vi "10_Scope.vi"(8 "error in (no error)":errorcluster) -> (0 "error out":errorcluster)   [LabVIEW 2014]
uses:
  SwabianInstruments.TimeTagger
panel:
  in  "Internal test signal":bool=TRUE
  in  "n_max_events":i32=1000
  in  "window_size":i64=10000000
  in  "trigger_channel":i32=1
  in  "event_channels":i32[](array[numeric])=[1, 2, 3]
  out "Scope":cluster{i64[], dbl[]}[](graph)
  # "This VI uses Scope measurement and plots test signal digital waveform.\n\nRun this VI to see the result."
  # "You can disable internal test signal\nand record your external signals."
  # "ps"
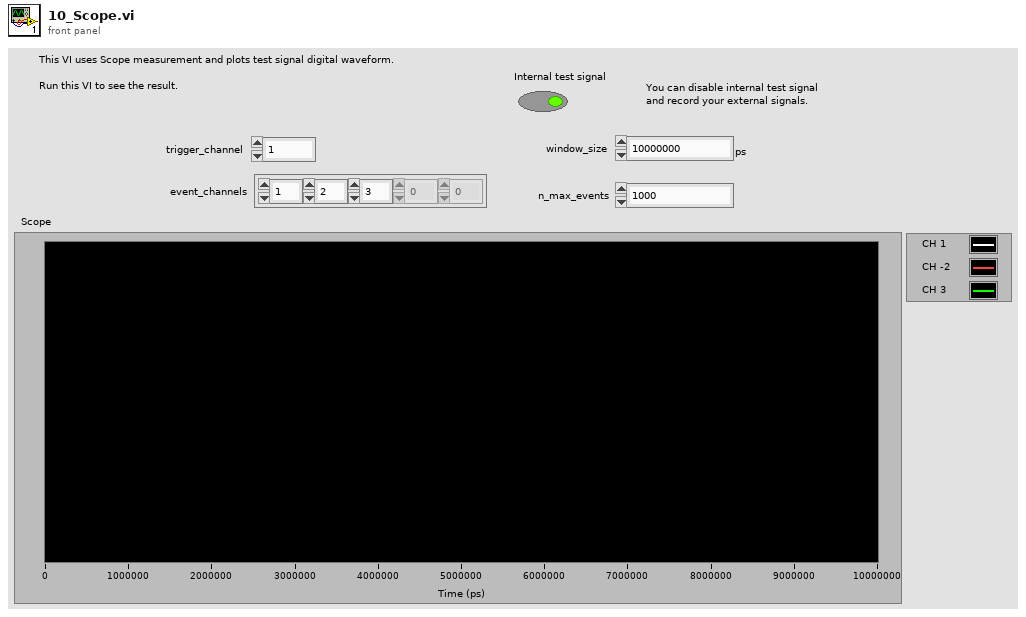
[diagram p1: front panel]
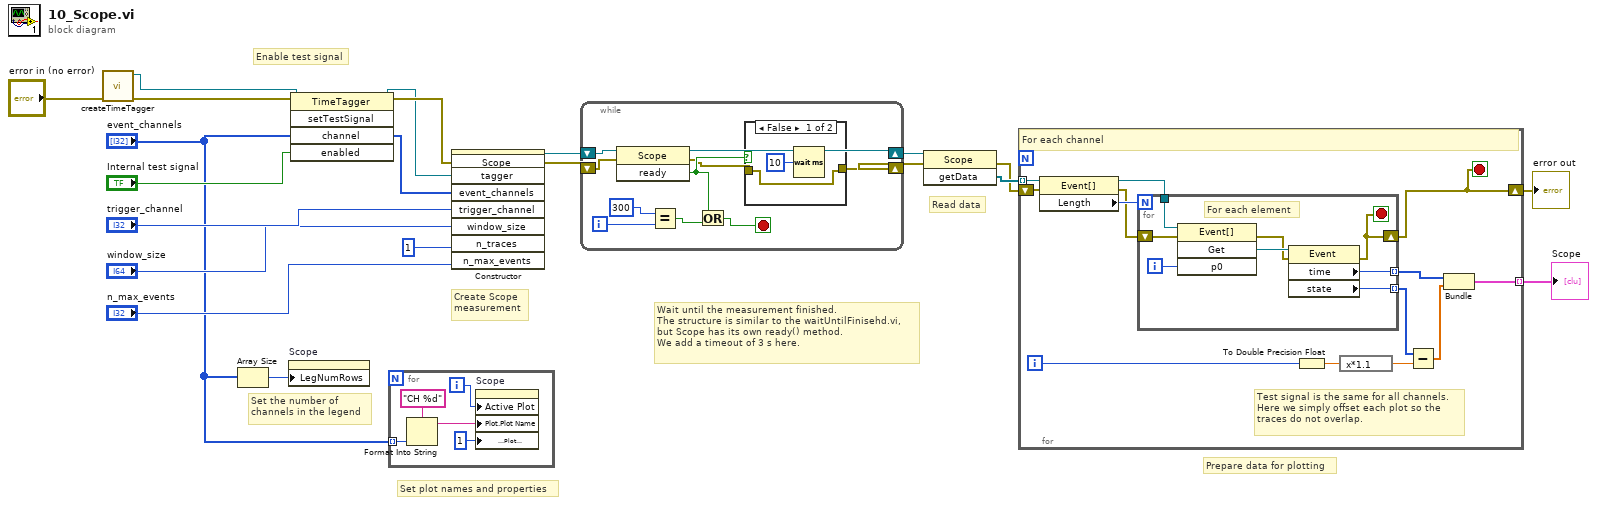
[diagram p0: block diagram]
diagram:
  # "Set plot names and properties"
  # "Set the number of \nchannels in the legend"
  # "Prepare data for plotting"
  # "Read data"
  # "Wait until the measurement finished.\nThe structure is similar to the waitUntilFinisehd.vi,\nbut Scope has its own ready() method.\nWe add a timeout of 3 s here."
  # "Create Scope \nmeasurement"
  # "Enable test signal"
  n1 = call "createTimeTagger.vi"("error in (no error)"="error in (no error)") -> ("error out"=w11:errorcluster, "TimeTagger ref out"=w12:refnum<k24>)  [unwired: 9 in]
  n2 = Array Size(array="event_channels") -> (size(s)=w8:i32)
  n3 = property on="Scope" class="XYGraph (strict)"("LegNumRows"=w8) -> ()  [unwired: 2 in, 2 out]
  n4 = invoke class="TimeTagger" method="setTestSignal"(reference=w12, error in=w11, "channel"="event_channels", "enabled"="Internal test signal") -> (reference out=w10:refnum<k24>, error out=w14:errorcluster, "channel"=w16:i32[])  [unwired: 1 in, 2 out]
  n5 = for {
    tunnel: "event_channels" -> [w26] mode=indexing
    i -> [w23]
    n6 = Format Into String(format string="CH %d", w26) -> (resulting string=w24:string)  [unwired: 2 in, 1 out]
    n7 = property on="Scope" class="XYGraph (strict)"("Active Plot"=w23, "Plot.Plot Name"=w24, "Plot.Plot Interpolation"=u8 1) -> ()  [unwired: 2 in, 2 out]
  }
  n8 = constructor class="Scope"(error in=w14, "tagger"=w10, "event_channels"=w16, "trigger_channel"="trigger_channel", "window_size"="window_size", "n_traces"=1, "n_max_events"="n_max_events") -> (reference out=w6:refnum<k24>, error out=w4:errorcluster)  [unwired: 2 in, 7 out]
  n9 = while {
    shift-right: [w34] -> w5
    shift-left: w6 -> [w36]
    shift-right: [w32] -> w3
    shift-left: w4 -> [w35]
    i -> [w30]
    stop <- w28 stop-if-true
    n10 = invoke class="Scope" method="ready"(reference=w36, error in=w35) -> (reference out=w34:refnum<k24>, error out=w31:errorcluster, "ready"=w33:bool)  [unwired: 1 in]
    n11 = Equal?(x=300 ("y"), y=w30) -> (x = y?=w29:bool)
    n12 = Or(x=w33, y=w29) -> (x .or. y?=w28:bool)
    n13 = case shown="False" w33 {
      tunnel: [w37 w39] -> w32
      tunnel: w31 -> [w37 w39]
      frame False {
        n14 = Wait (ms)(milliseconds to wait=u32 10) -> ()  [unwired: 1 out]
      }
      frame True {
      }
    }
  }
  n15 = invoke class="Scope" method="getData"(reference=w5, error in=w3) -> (error out=w13:errorcluster, "getData"=w17:refnum<k24>[])  [unwired: 1 in, 1 out]
  n16 = for {
    tunnel: w17 -> [w51] mode=indexing
    tunnel: [w48] -> w7 mode=indexing
    shift-right: [w44] -> w2
    shift-left: w13 -> [w46]
    i -> [w42]
    stop <- w44 stop-if-true
    # "Test signal is the same for all channels. \nHere we simply offset each plot so the\ntraces do not overlap."
    # "For each channel"
    n17 = property class="Event[]"(reference=w51, error in=w46) -> (reference out=w47:refnum<k24>, error out=w45:errorcluster, "Length"=w52:i32)
    n18 = for {
      N: w52 -> [_]
      tunnel: w47 -> [w60]
      tunnel: [w57] -> w50 mode=indexing
      tunnel: [w56] -> w49 mode=indexing
      shift-right: [w53] -> w44
      shift-left: w45 -> [w55]
      i -> [w59]
      stop <- w53 stop-if-true
      # "For each element"
      n19 = invoke class="Event[]" method="Get"(reference=w60, error in=w55, "p0"=w59) -> (error out=w54:errorcluster, "Get"=w58:refnum<k24>)  [unwired: 1 in, 2 out]
      n20 = property class="Event"(reference=w58, error in=w54) -> (error out=w53:errorcluster, "time"=w57:i64, "state"=w56:i32)  [unwired: 1 out]
    }
    n21 = To Double Precision Float(number=w42) -> (double precision float=w40:dbl)
    n22 = expression code="x*1.1"(w40) -> (w41:dbl)
    n23 = Subtract(x=w49, y=w41) -> (x-y=w43:dbl[])
    n24 = Bundle(w50, w43) -> (w48:cluster{i64[], dbl[]})  [unwired: 1 in]
  }
  "Scope" <- w7
  "error out" <- w2
